vi "Create All Message Queues.vi"(8 "error in (no error)":errorcluster, 11 "Message Queue Name (\"\")":string) -> (0 "error out":errorcluster, 3 "Message Queues out":T1)   [LabVIEW 2020, in "User Interface Utilities.lvlib" / "Message Queue.lvlib"]
doc: "This VI creates and initializes all the message queues for your application. If your application requires more than one message queue, right-click the \"Message Queues\" constant above and select Open Type Def. Add the new Message Queue(s) to the type definition, then initialize them in this VI."
uses:
  Message Queue.lvlib
  All Message Queues.ctl
  Message.ctl
  Enqueue Message (Single).vi
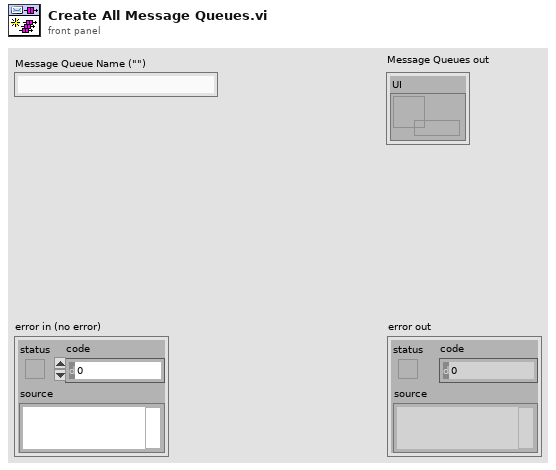
[diagram p1: front panel]
types:
  T1 = typedef "User Interface Utilities.lvlib/Message Queue.lvlib/All Message Queues.ctl" = cluster{"UI":refnum<queue>}
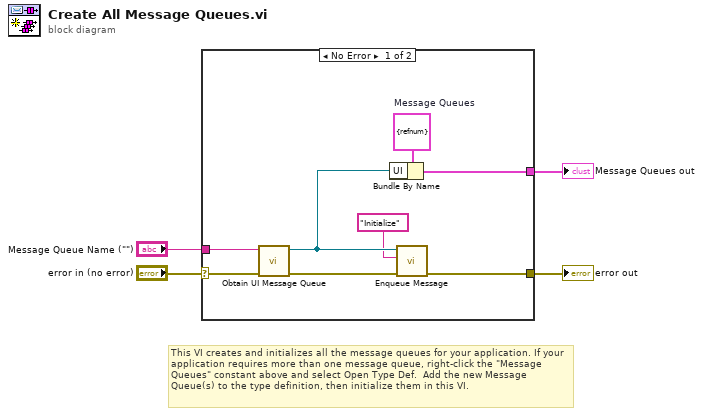
[diagram p0: block diagram]
diagram:
  # "This VI creates and initializes all the message queues for your application. If your application requires more than one message queue, right-click the \"Message Queues\" constant above and select Open Type Def.  Add the new Message Queue(s) to the type definition, then initialize them in this VI."
  n1 = case shown="No Error" "error in (no error)" {
    selector: "error in (no error)" -> [w9 w13]
    tunnel: [w12 w13] -> w4
    tunnel: [w10 _] -> w3
    tunnel: "Message Queue Name (\"\")" -> [w5 _]
    frame No Error {
      w11 = T1 {"UI"=refnum}  # Message Queues
      n2 = call "Obtain UI Message Queue.vi"("error in (no error)"=w9, "Name (unnamed)"=w5) -> ("error out"=w8:errorcluster, "Message Queue"=w7:refnum<queue>)  [unwired: 8 in]
      n3 = Bundle By Name(cluster=w11, "UI"=w7) -> (w10:T1)
      n4 = call-poly "Enqueue Message.vi"("error in (no error)"=w8, "Action"="Initialize", "Message Queue"=w7) -> ("error out"=w12:errorcluster)  [unwired: 7 in, 1 out]
    }
    frame Error {
    }
  }
  "Message Queues out" <- w3
  "error out" <- w4
